vi "Test Session.vi"() -> ()   [LabVIEW 2020]
uses:
  <vilib>/Utility/lvfile.llb/FT_FileTypes.ctl
  LabVIEW Project File/LabVIEW Project File.lvclass
  LabVIEW File/LabVIEW File.lvclass
  \\Mac\Home/JKI/GitHub/save-for-previous-labview-version/source/File/File.lvclass/File.lvclass
  Session/Session.lvclass
  <vilib>/Utility/lvfile.llb/NI_FileType.lvlib
  File/File.lvclass/File.lvclass
panel:
  in  "Save for Previous":bool
  out "Actual Root Source Folder of Export":path
  out "Different Drives?":bool
  out "error out":errorcluster
  out "Destination Folder":path
  out "Current Project":path
  in  "Files":i32(listbox)
  in  "LabVIEW Version":string
  in  "Source Folder":path
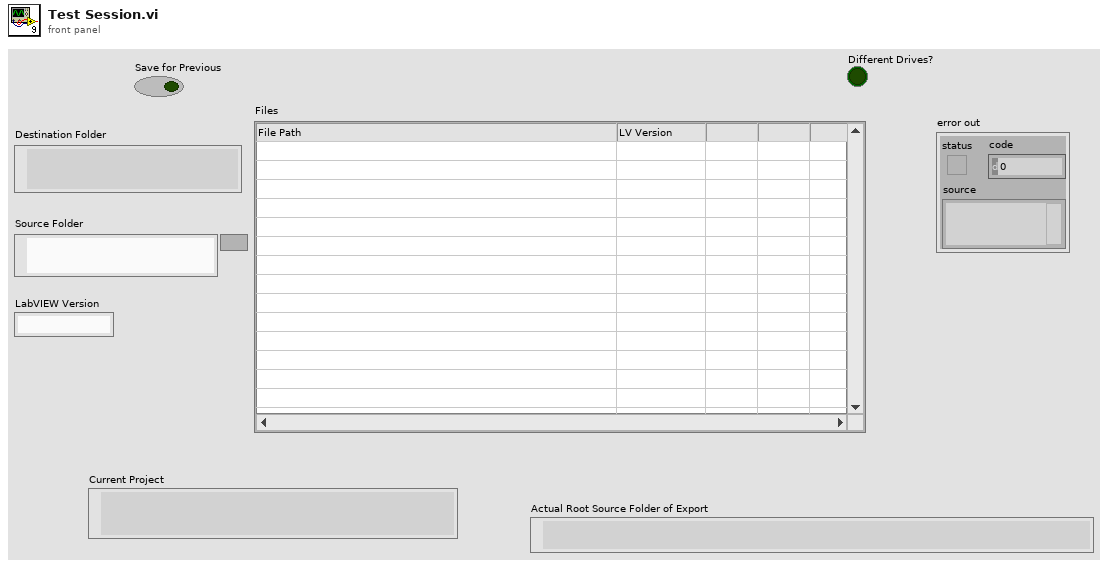
[diagram p1: front panel]
types:
  T1 = typedef "NI_FileType.lvlib/FT_FileTypes.ctl" = enum32{"Invalid file/path", "Unknown type", "Instrument", "Control", "Polymorphic VI", "Project", "Library", "LVClass", "XControl", "XNode", "CIN", "Run-time menu", "Palette menu", "LLB", "Shortcut", "Directory", "Class Private Data Control", "Statechart", "MathScript .m file", "Ladder Diagram", "LVLibp"}
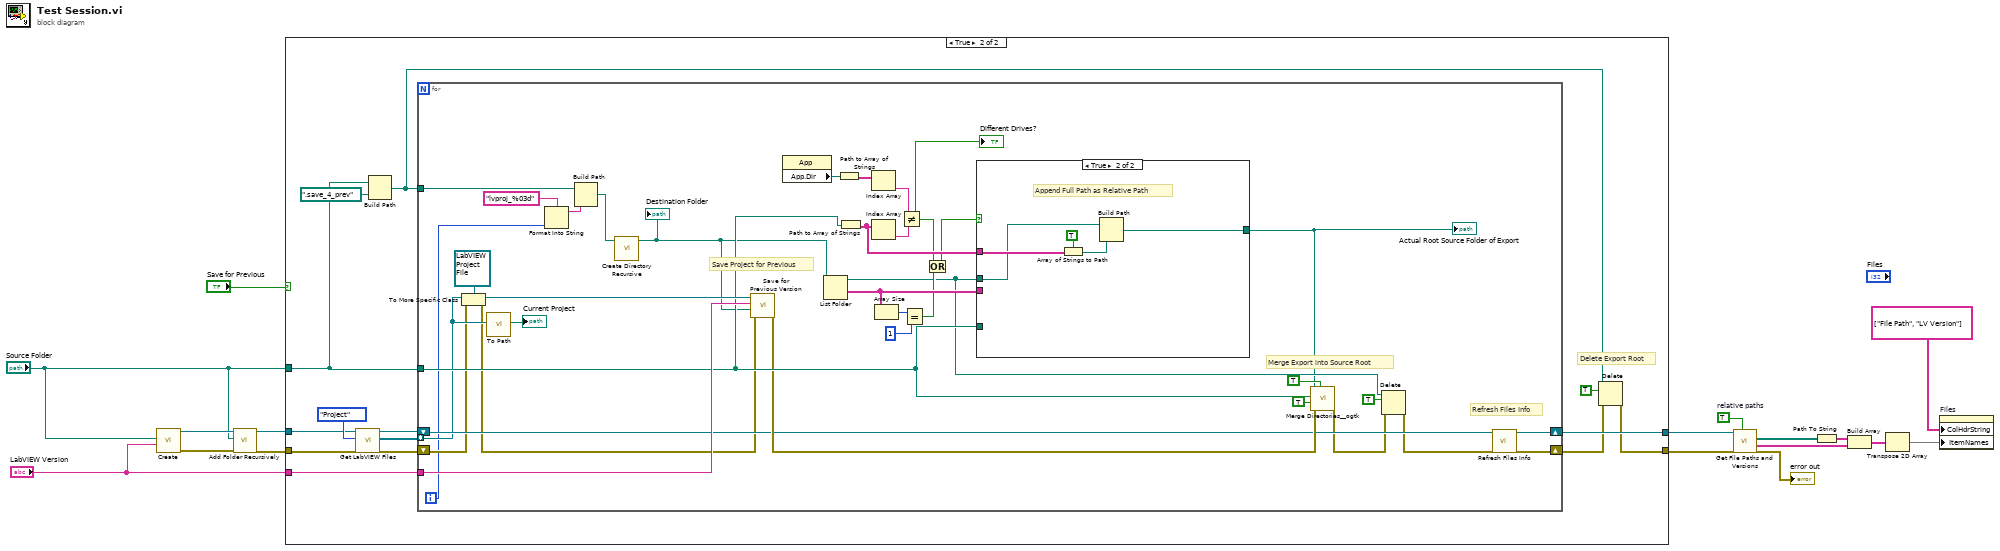
[diagram p0: block diagram]
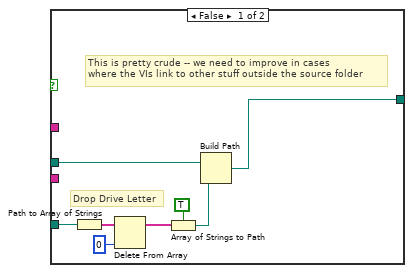
[diagram p3: hidden frame]
diagram:
  w9 = TRUE  # relative paths
  n1 = call "Create.vi"("LabVIEW Version"="LabVIEW Version", "Source Folder"="Source Folder") -> ("error out"=w16:errorcluster, "Session out"=w17:refnum<class "Session.lvclass">)  [unwired: 8 in]
  n2 = call "Add Folder Recursively.vi"("error in (no error)"=w16, "Folder"="Source Folder", "Session in"=w17) -> ("error out"=w7:errorcluster, "Session out"=w8:refnum<class "Session.lvclass">)  [unwired: 7 in]
  n3 = case shown="True" "Save for Previous" {
    tunnel: w8 -> [w19 w32]
    tunnel: w7 -> [w18 w31]
    tunnel: "LabVIEW Version" -> [_ w29]
    tunnel: [w19 w26] -> w4
    tunnel: "Source Folder" -> [_ w25]
    tunnel: [w18 w21] -> w2
    frame False {
    }
    frame True {
      # "Delete Export Root"
      n4 = call "Get LabVIEW Files.vi"("error in (no error)"=w31, "LabVIEW File Type"=FT_FileTypes."Project", "Session in"=w32) -> ("error out"=w28:errorcluster, "LabVIEW Files"=w30:refnum<class "LabVIEW File.lvclass">[], "Session out"=w27:refnum<class "Session.lvclass">)  [unwired: 6 in]
      n5 = Build Path(base path=w25, name or relative path=path ".save_4_prev") -> (appended path=w20:path)
      n6 = for {
        tunnel: w30 -> [w43] mode=indexing
        tunnel: w29 -> [w66]
        tunnel: w25 -> [w60]
        shift-right: [w54] -> w22
        shift-left: w28 -> [w42]
        shift-right: [w55] -> w26
        shift-left: w27 -> [w56]
        tunnel: w20 -> [w36]
        i -> [w39]
        # "Merge Export into Source Root"
        # "Refresh Files Info"
        # "Save Project for Previous"
        n7 = To More Specific Class(target class=refnum<class "LabVIEW Project File.lvclass"> refnum ("LabVIEW Project File in"), reference=w43, error in=w42) -> (specific class reference=w67:refnum<class "LabVIEW Project File.lvclass">, error out=w41:errorcluster)
        n8 = call "To Path.vi"("File in"=w43) -> ("Path out"=→"Current Project":path)  [unwired: 10 in]
        n9 = Format Into String(format string="lvproj_%03d", w39) -> (resulting string=w37:string)  [unwired: 2 in, 1 out]
        n10 = Build Path(base path=w36, name or relative path=w37) -> (appended path=w35:path)
        n11 = call <vilib>:"Create Directory Recursive.vi"("directory"=w35) -> ("directory copy"=w34:path)  [unwired: 4 in, 2 out]
        "Destination Folder" <- w34
        n12 = call-dynamic "Save for Previous Version.vi"("error in (no error)"=w41, "Destination Folder (\"\": In Place)"=w34, "LabVIEW Version"=w66, "LabVIEW Project File in"=w67) -> ("error out"=w57:errorcluster)  [unwired: 4 in, 3 out]
        n13 = property class="App"() -> ("App.Dir"=w65:path)  [unwired: 2 in, 2 out]
        n14 = List Folder(path=w34) -> (path out=w47:path, folder names=w53:string[])  [unwired: 3 in, 2 out]
        n15 = Path to Array of Strings(0:w65) -> (2:w61:string[])  [unwired: 1 out]
        n16 = Path to Array of Strings(0:w60) -> (2:w62:string[])  [unwired: 1 out]
        n17 = Index Array(array=w61) -> (element=w64:string)  [unwired: 1 in]
        n18 = Index Array(array=w62) -> (element=w63:string)  [unwired: 1 in]
        n19 = Array Size(array=w53) -> (size(s)=w52:i32)
        n20 = Not Equal?(x=w64, y=w63) -> (x != y?=w49:bool)
        "Different Drives?" <- w49
        n21 = Equal?(x=w52, y=1) -> (x = y?=w50:bool)
        n22 = Or(x=w49, y=w50) -> (x .or. y?=w48:bool)
        n23 = case shown="True" w48 {
          tunnel: w62 -> [_ w82]
          tunnel: w47 -> [w71 w79]
          tunnel: [w70 w78] -> w40
          tunnel: w53 -> [_ _]
          tunnel: w60 -> [w77 _]
          frame False {
            # "This is pretty crude -- we need to improve in cases\nwhere the VIs link to other stuff outside the source folder"
            # "Drop Drive Letter"
            n24 = Path to Array of Strings(0:w77) -> (2:w76:string[])  [unwired: 1 out]
            n25 = Delete From Array(array=w76, index=0) -> (array with subset deleted=w72:string[])  [unwired: 1 in, 1 out]
            n26 = Array of Strings to Path(0:w72, 1:TRUE ("relative")) -> (2:w73:path)
            n27 = Build Path(base path=w71, name or relative path=w73) -> (appended path=w70:path)
          }
          frame True {
            # "Append Full Path as Relative Path"
            n28 = Array of Strings to Path(0:w82, 1:TRUE ("relative")) -> (2:w80:path)
            n29 = Build Path(base path=w79, name or relative path=w80) -> (appended path=w78:path)
          }
        }
        "Actual Root Source Folder of Export" <- w40
        n30 = call <userlib>:"Merge Directories__ogtk.vi"("Delete Source? (FALSE)"=TRUE, "error in (no error)"=w57, "Overwrite Existing Files? (FALSE)"=TRUE, "target directory path"=w60, "source directory path"=w40) -> ("error out"=w45:errorcluster)  [unwired: 5 in, 1 out]
        n31 = Delete(path (use dialog)=w47, entire hierarchy (F)=TRUE, error in=w45) -> (error out=w44:errorcluster)  [unwired: 2 in, 2 out]
        n32 = call "Refresh Files Info.vi"("error in (no error)"=w44, "Session in"=w56) -> ("error out"=w54:errorcluster, "Session out"=w55:refnum<class "Session.lvclass">)  [unwired: 8 in]
      }
      n33 = Delete(path (use dialog)=w20, entire hierarchy (F)=TRUE, error in=w22) -> (error out=w21:errorcluster)  [unwired: 2 in, 2 out]
    }
  }
  n34 = call "Get File Paths and Versions.vi"("relative paths? (F: Absolute)"=w9, "error in (no error)"=w2, "Session in"=w4) -> ("error out"=→"error out":errorcluster, "Versions"=w12:string[], "File Paths"=w14:path[])  [unwired: 5 in, 1 out]
  n35 = Path To String(path=w14) -> (string=w13:string[])
  n36 = Build Array(w13, w12) -> (w11:string[][])
  n37 = Transpose 2D Array(2D array=w11) -> (transposed array=w10:string[][])
  n38 = property on="Files" class="MCListbox (strict)"("ColHdrString"=string[] ["File Path", "LV Version"] ("Row Header Strings[]"), "ItemNames"=w10) -> ()  [unwired: 2 in, 2 out]
